vi "LoadClassFromFile.vi"(8 "error in (no error)":errorcluster, 10 "class path":path, 11 "reference in":refnum<class "BaseObject.lvclass">) -> (0 "error out":errorcluster, 3 "reference out":refnum<class "BaseObject.lvclass">)   [LabVIEW 2014, in "BaseClasses.lvlib" / "BaseObject.lvclass"]
uses:
  BaseObject.lvclass
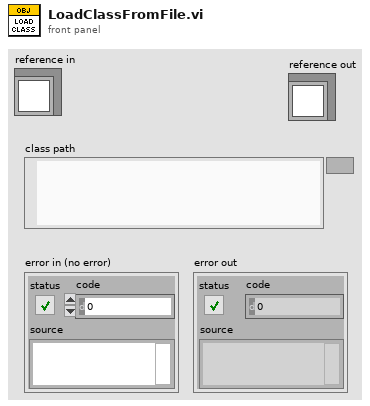
[diagram p1: front panel]
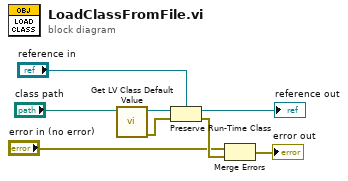
[diagram p0: block diagram]
diagram:
  n1 = call <vilib>:"Get LV Class Default Value.vi"("class path"="class path") -> ("error out"=w6:errorcluster, "object"=w7:refnum<class>)  [unwired: 9 in]
  n2 = Preserve Run-Time Class(object in=w7, error in=w6, 2:"reference in") -> (object out=→"reference out":refnum<class "BaseObject.lvclass">, error out=w5:errorcluster)
  n3 = Merge Errors("error in (no error)", w5) -> (→"error out":errorcluster)
